vi "AlliGator Get Image Binning String.vi"(8 "Error In":errorcluster, 11 "Image Binning Options":T1 {"Y Bin" min=1; "X Bin" min=1}) -> (0 "Error Out":errorcluster, 3 "String":string)   [LabVIEW 2021, in "AlliGator Files.lvlib"]
doc: "Get image binning options string."
uses:
  AlliGator Files.lvlib
  Source Image/AlliGator Image Binning Options.ctl
  Source Image/AlliGator Source Image.lvlib
panel:
  # "see the AlliGator License on the block diagram (Ctrl+E or Window:Show Block Diagram)"
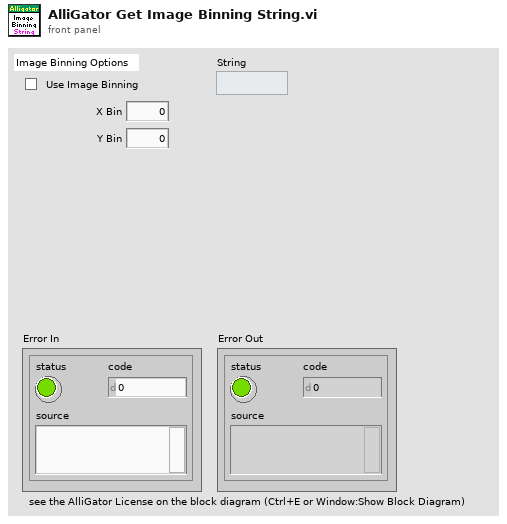
[diagram p1: front panel]
types:
  T1 = typedef "AlliGator Source Image.lvlib/AlliGator Image Binning Options.ctl" = cluster{"Use Image Binning":bool, "X Bin":i32, "Y Bin":i32}
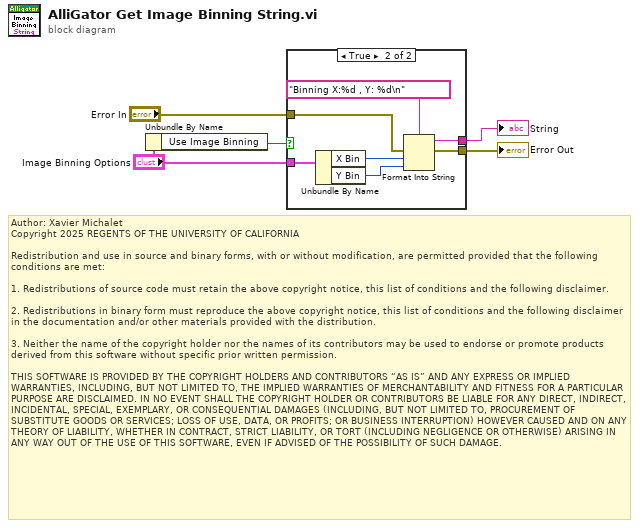
[diagram p0: block diagram]
diagram:
  # "Author: Xavier Michalet\nCopyright 2025 REGENTS OF THE UNIVERSITY OF CALIFORNIA\n\nRedistribution and use in source and binary forms, with or without modification, are permitted provided that the following conditions are met:\n\n1. Redistributions of source code must retain the above copyright notice, this list of conditions and the following disclaimer.\n\n2. Redistributions in binary form must reproduce the above copyright notice, this list of conditions and the following disclaimer in the documentation and/or other materials provided with the distribution.\n\n3. Neither the name of the copyright holder nor the names of its contributors may be used to endorse or promote products derived from this software without specific prior written permission.\n\nTHIS SOFTWARE IS PROVIDED BY THE COPYRIGHT HOLDERS AND CONTRIBUTORS “AS IS” AND ANY EXPRESS OR IMPLIED WARRANTIES, INCLUDING, BUT NOT LIMITED TO, THE IMPLIED WARRANTIES OF MERCHANTABILITY AND FITNESS FOR A PARTICULAR PURPOSE ARE DISCLAIMED. IN NO EVENT SHALL THE COPYRIGHT HOLDER OR CONTRIBUTORS BE LIABLE FOR ANY DIRECT, INDIRECT, INCIDENTAL, SPECIAL, EXEMPLARY, OR CONSEQUENTIAL DAMAGES (INCLUDING, BUT NOT LIMITED TO, PROCUREMENT OF SUBSTITUTE GOODS OR SERVICES; LOSS OF USE, DATA, OR PROFITS; OR BUSINESS INTERRUPTION) HOWEVER CAUSED AND ON ANY THEORY OF LIABILITY, WHETHER IN CONTRACT, STRICT LIABILITY, OR TORT (INCLUDING NEGLIGENCE OR OTHERWISE) ARISING IN ANY WAY OUT OF THE USE OF THIS SOFTWARE, EVEN IF ADVISED OF THE POSSIBILITY OF SUCH DAMAGE."
  n1 = Unbundle By Name("Image Binning Options") -> ("Use Image Binning"=w3:bool)
  n2 = case shown="True" w3 {
    tunnel: [_ w13] -> w5
    tunnel: "Image Binning Options" -> [_ w9]
    tunnel: "Error In" -> [w6 w12]
    tunnel: [w6 w11] -> w1
    frame False {
    }
    frame True {
      n3 = Unbundle By Name(w9) -> ("X Bin"=w8:i32, "Y Bin"=w7:i32)
      n4 = Format Into String(format string="Binning X:%d , Y: %d\n", error in=w12, w8, w7) -> (resulting string=w13:string, error out=w11:errorcluster)  [unwired: 1 in]
    }
  }
  "String" <- w5
  "Error Out" <- w1
